vi "Update Configuration.vi"(8 "error in (no error)":errorcluster, 11 "CIFPlugin in":refnum<class "Template_Plugin.lvclass">) -> (0 "error out":errorcluster, 3 "CIFPlugin out":refnum<class "Template_Plugin.lvclass">)   [LabVIEW 2021, in "Template_Plugin.lvclass"]
uses:
  Template_Plugin.lvclass
  C:/Program Files/National Instruments/LabVIEW 2021/vi.lib/CIF Foundation/CIF Core/CIFCore/Class/CIFCorePlugin.lvclass
  <vilib>/CIF Foundation/CIF Core/CIFCore/Class/CIFCorePlugin.lvclass/CIFCorePlugin.ctl
  Template_Plugin.lvclass/Template_Plugin.ctl
  <vilib>/CIF Foundation/CIF Core/CIFCore/Class/Accessors/Write Configuration Change.vi
  <vilib>/CIF Foundation/CIF Core/CIFCore/Class/CIFCorePlugin.lvclass
  D:/dev/Plugins/Template/src/Source/CIF/Plugin Generator/Template/Class/Template_Plugin.lvclass
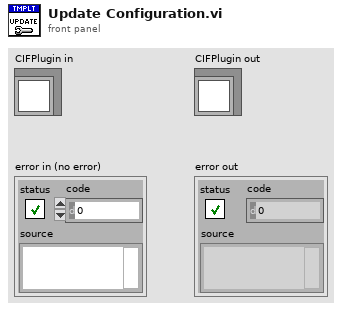
[diagram p1: front panel]
types:
  T1 = typedef "Template_Common.lvlib/Configuration.ctl" = cluster{"Common":T2, "Step":u64}
  T2 = typedef "CIFCoreCommon.lvlib/Common Plugin Configuration.ctl" = cluster{"Period (s)":dbl, "Offset (us)":i32, "Priority":i32, "Processor":i32, "External Clock":T3}
  T3 = typedef "CIFCoreCommon.lvlib/External Clock Config.ctl" = cluster{"ClockID":u8, "Clock Name":string, "Publish Clock":bool, "Convert Data Timestamps":bool, "Plugin Timing Source":bool}
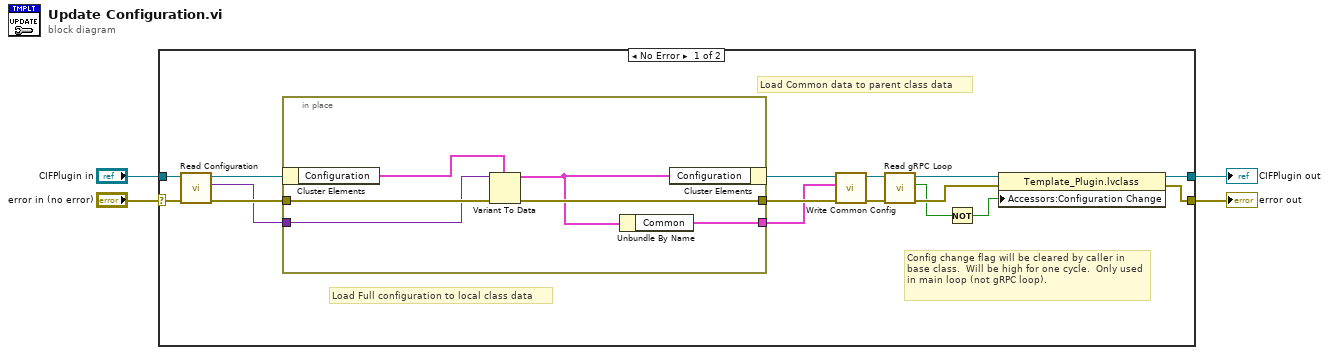
[diagram p0: block diagram]
diagram:
  n1 = case shown="No Error" "error in (no error)" {
    selector: "error in (no error)" -> [w16 w27]
    tunnel: "CIFPlugin in" -> [w17 w28]
    tunnel: [w12 w28] -> w1
    tunnel: [w11 w27] -> w3
    frame No Error {
      # "Config change flag will be cleared by caller in base class.  Will be high for one cycle.  Only used in main loop (not gRPC loop)."
      # "Load Common data to parent class data"
      # "Load Full configuration to local class data"
      n2 = call <vilib>:"Read Configuration.vi"("error in"=w16, "CIFCorePlugin in"=w17) -> ("error out"=w15:errorcluster, "Configuration Data"=w14:variant, "CIFCorePlugin out"=w13:refnum<class "Template_Plugin.lvclass">)  [unwired: 7 in]
      n3 = in-place {
        in-place-border: [w26] -> w20
        in-place-border: w15 -> [w25]
        in-place-border: w14 -> [w24]
        in-place-border: [w22] -> w19
        n4 = in-place-cluster #1(w13) -> ("Configuration"=w23:T1)
        n5 = Variant To Data(error in=w25, type=w23, Variant=w24) -> (data=w21:T1, error out=w26:errorcluster)
        n6 = Unbundle By Name(w21) -> ("Common"=w22:T2)
        n7 = in-place-cluster #1("Configuration"=w21) -> (w18:refnum<class "Template_Plugin.lvclass">)
      }
      n8 = call <vilib>:"Write Common Config.vi"("error in (no error)"=w20, "Common"=w19, "CIFTemplateNode in"=w18) -> ("error out"=w9:errorcluster, "CIFTemplateNode out"=w10:refnum<class "Template_Plugin.lvclass">)  [unwired: 7 in]
      n9 = call <vilib>:"Read gRPC Loop.vi"("error in (no error)"=w9, "CIFCorePlugin in"=w10) -> ("error out"=w7:errorcluster, "gRPC Loop"=w5:bool, "CIFCorePlugin out"=w8:refnum<class "Template_Plugin.lvclass">)  [unwired: 7 in]
      n10 = Not(x=w5) -> (.not. x?=w6:bool)
      n11 = property class="Template_Plugin.lvclass"(reference=w8, error in=w7, "Accessors:Configuration Change"=w6) -> (reference out=w12:refnum<class "Template_Plugin.lvclass">, error out=w11:errorcluster)
    }
    frame Error {
    }
  }
  "error out" <- w3
  "CIFPlugin out" <- w1
